vi "Translate Core.vi"(8 "error in (no error)":errorcluster, 10 "Translation":T1, 11 "Shape in":refnum<class "Shape.lvclass">) -> (0 "error out":errorcluster, 3 "Shape out":refnum<class "Shape.lvclass">)   [LabVIEW 2017, in "LV Image Editor Framework.lvlib" / "Shape.lvclass"]
uses:
  Shape.lvclass
  <vilib>/Utility/miscctls.llb/LVPoint32TypeDef.ctl
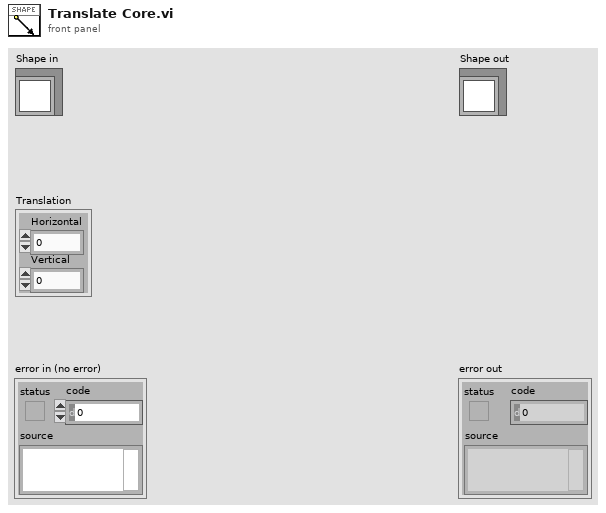
[diagram p1: front panel]
types:
  T1 = typedef "LVPoint32TypeDef.ctl" = cluster{"Horizontal":i32, "Vertical":i32}
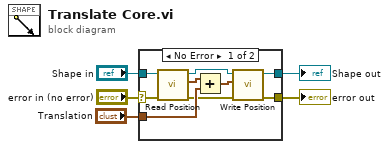
[diagram p0: block diagram]
diagram:
  n1 = case shown="No Error" "error in (no error)" {
    selector: "error in (no error)" -> [w6 w16]
    tunnel: [w8 w16] -> w4
    tunnel: [w9 w15] -> w2
    tunnel: "Shape in" -> [w13 w15]
    tunnel: "Translation" -> [w14 _]
    frame No Error {
      n2 = call-dynamic "Read Position.vi"("error in (no error)"=w6, "Shape in"=w13) -> ("error out"=w7:errorcluster, "Position"=w11:cluster{"Left":i32, "Top":i32}, "Shape out"=w12:refnum<class "Shape.lvclass">)  [unwired: 7 in]
      n3 = Add(x=w11, y=w14) -> (x+y=w10:T1)
      n4 = call-dynamic "Write Position.vi"("error in (no error)"=w7, "Position"=w10, "Shape in"=w12) -> ("error out"=w8:errorcluster, "Shape out"=w9:refnum<class "Shape.lvclass">)  [unwired: 7 in]
    }
    frame Error {
    }
  }
  "error out" <- w4
  "Shape out" <- w2
